vi "calculate histogram.vi"(6 "channel no.":i32, 7 "Image Ctrl Ref (as generic class)":refnum<vi>, 8 "Image Array":i16[][](array[numeric]), 11 "Image":T1) -> ()   [LabVIEW 2012]
uses:
  <vilib>/vision/Image Controls.llb/IMAQ Image.ctl
  GFG/GFGfpRefGet.vi
  GFG/GFGbooleanGet.vi
  <vilib>/vision/NI_Vision_Development_Module.lvlib
  GFG/GFG library.lvlib
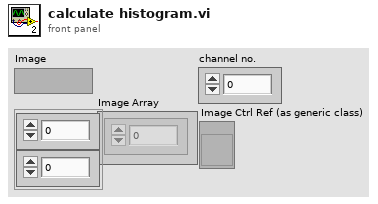
[diagram p1: front panel]
types:
  T1 = typedef "IMAQ Image.ctl" = refnum<image>
  T2 = cluster{"Starting Value":sgl, "Incremental Value":sgl, "Histogram":u32[]}
  T3 = cluster{"WaveformChartRef":refnum<vi>, "DigitalRef":refnum<vi>, "ArrayRef":refnum<vi>, "TabControlRef":refnum<vi>, "EnumRef":refnum<vi>, "RingRef":refnum<vi>, "BooleanRef":refnum<vi>, "KnobRef":refnum<vi>, "SlideRef":refnum<vi>, "PathRef":refnum<vi>, "StringRef":refnum<vi>, "ComboBox":refnum<vi>, "WaveformGraphRef":refnum<vi>}
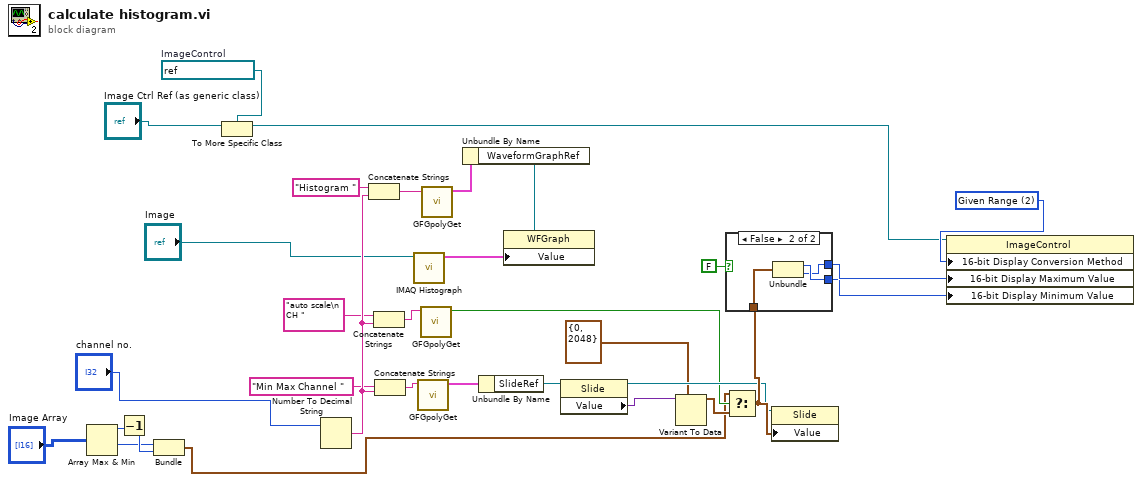
[diagram p0: block diagram]
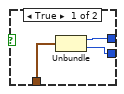
[diagram p2: hidden frame]
diagram:
  w5 = refnum<vi> refnum  # ImageControl
  w14 = u32 2 items=["Full Dynamic", "Downshift", "Given Range", "90% Dynamic", "Given Percent Range"] ("16-bit Display Mapping:Conversion Method")
  n1 = Array Max & Min(array="Image Array") -> (max value=w10:i16, min value=w11:i16)  [unwired: 2 out]
  n2 = Decrement(x=w10) -> (x-1=w12:i16)
  n3 = Bundle(w11, w12) -> (w9:cluster{i16, i16})  [unwired: 1 in]
  n4 = To More Specific Class(target class=w5, reference="Image Ctrl Ref (as generic class)") -> (specific class reference=w4:refnum<vi>)  [unwired: 1 in, 1 out]
  n5 = Number To Decimal String(number="channel no.") -> (decimal integer string=w24:string)  [unwired: 1 in]
  n6 = Concatenate Strings("Histogram " ("string"), w24) -> (w18:string)
  n7 = Concatenate Strings("auto scale\n      CH " ("Variable Name in"), w24) -> (w21:string)
  n8 = Concatenate Strings("Min Max Channel " ("Variable Name in"), w24) -> (w31:string)
  n9 = call "IMAQ Histograph"("Image"="Image") -> ("Histogram Graph"=w15:T2)  [unwired: 7 in, 3 out]
  n10 = call-poly "GFGpolyGet.vi"("Variable Name in"=w31) -> ("output cluster"=w22:T3)  [unwired: 9 in, 1 out]
  n11 = call-poly "GFGpolyGet.vi"("Variable Name in"=w21) -> ("Boolean"=w28:bool)  [unwired: 10 in]
  n12 = call-poly "GFGpolyGet.vi"("Variable Name in"=w18) -> ("output cluster"=w17:T3)  [unwired: 9 in, 1 out]
  n13 = Unbundle By Name(w17) -> ("WaveformGraphRef"=w16:refnum<vi>)
  n14 = Unbundle By Name(w22) -> ("SlideRef"=w25:refnum<vi>)
  n15 = property class="WFGraph"(reference=w16, "Value"=w15) -> ()  [unwired: 1 in, 2 out]
  n16 = property class="Slide"(reference=w25) -> (reference out=w30:refnum<vi>, "Value"=w26:variant)  [unwired: 1 in, 1 out]
  n17 = Variant To Data(type=cluster{i32, i32} {0, 2048} ("channel1"), Variant=w26) -> (data=w29:cluster{i32, i32})  [unwired: 1 in, 1 out]
  n18 = Select(t=w9, s=w28, f=w29) -> (s? t:f=w32:cluster{i32, i32})
  n19 = case shown="False" FALSE {
    tunnel: w32 -> [w35 w38]
    tunnel: [w34 w36] -> w3
    tunnel: [w33 w37] -> w2
    frame True {
      n20 = Unbundle(w35) -> (w34:i32, w33:i32)
    }
    frame False {
      n21 = Unbundle(w38) -> (w37:i32, w36:i32)
    }
  }
  n22 = property class="Slide"(reference=w30, "Value"=w32) -> ()  [unwired: 1 in, 2 out]
  n23 = property class="ImageControl"(reference=w4, "16-bit Display Conversion Method"=w14, "16-bit Display Maximum Value"=w3, "16-bit Display Minimum Value"=w2) -> ()  [unwired: 1 in, 2 out]
